vi "SwapTimeState.vi"(10 "Old cluster":T1, 11 "New cluster":T1) -> (3 "Cluster out":T1)   [LabVIEW 2018]
doc: "Scambia i valori dell'old cluster con i valori del nuovo cluster e restituisce il risultato."
uses:
  TimeCluster.ctl
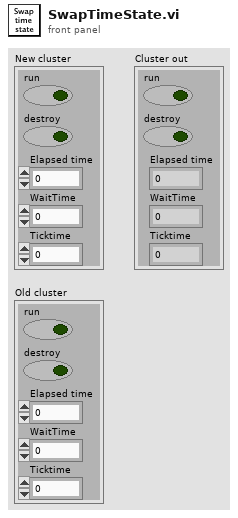
[diagram p1: front panel]
types:
  T1 = typedef "TimeCluster.ctl" = cluster{"run":bool, "destroy":bool, "Elapsed time":i32, "WaitTime":i32, "Ticktime":i32}
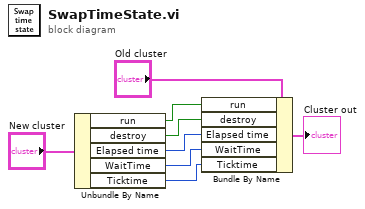
[diagram p0: block diagram]
diagram:
  n1 = Unbundle By Name("New cluster") -> ("run"=w5:bool, "destroy"=w4:bool, "Elapsed time"=w3:i32, "WaitTime"=w2:i32, "Ticktime"=w1:i32)
  n2 = Bundle By Name(cluster="Old cluster", "run"=w5, "destroy"=w4, "Elapsed time"=w3, "WaitTime"=w2, "Ticktime"=w1) -> (→"Cluster out":T1)
